vi "ISOP camera console.vi"() -> ()   [LabVIEW 2024]
uses:
  Global variables/global for picoscope.vi
  Global variables/Global for awg.vi
  Global variables/Global 1.vi
  Global variables/Global calib.vi
  Global variables/filepath global variable.vi
  <vilib>/Utility/file.llb/Write Delimited Spreadsheet (DBL).vi
  RIGOL DG4000 Series/RIGOL DG4000 Series.lvlib
  old LabVIEW files/labview_Mikami/Teledyne LeCroy WaveStation/Teledyne LeCroy WaveStation.lvlib
panel:
  in  "AOD exc λ2 [nm]":dbl=560.0
  in  "g2 monitor coeff [V/mdeg] am2":dbl=0.41
  in  "g1(SCAPE) phase":dbl=347.99999999999994
  in  "round-trip":bool
  in  "force":bool
  in  "vol rate [Hz]":dbl=123.00123001230013
  in  "vol period [s]":dbl=0.00813
  in  "xy pixsize [um]":dbl=0.4094999999999999
  in  "latest":bool=TRUE
  in  "g1 fit coeffs":path=path "E:/g1fitcalib/20241212-124823.g1fit"
  in  "?":bool
  in  "fit coeffs":dbl[][](array[numeric])=[[0.0003442175414953786, -6.156938994794033e-08], [-0.00558042162015375, 7.101515384977181e-07]]
  out "g2 ofst for calib":dbl=-0.1319999999999999 format="%_3g"
  in  "target freq for monitor":dbl=5.0
  in  "load config":bool
  in  "load config filepath":path
  in  "config filename":string
  in  "save config":bool
  in  "stop 2":bool
  in  "g1(scape)on/off":bool=TRUE
  in  "g1(SCAPE) p coeff":dbl format="%_4g"
  out "RIGOL name":refnum<visa-resource-name>="USB0::0x1AB1::0x0641::DG4E223801593::INSTR"
  in  "g1 (SCAPE) wvfm ofst [V]":dbl=1.0 format="%_4g"
  in  "g1 (SCAPE) gain adjust":dbl=1.0 format="%_4g"
  in  "g1 (SCAPE) gap adjust":dbl=1.0 format="%_4g"
  in  "rec with max freq":bool
  in  "target freq [Hz] for rec":dbl=10.0
  out "calib":bool
  in  "Config":T1={"Clock source"=enum."1200 MHz", "Active channel"=enum."Four channel", "Trigger direction"=enum."Positive (Rising edge)", "Trigger mode"=enum."Per trigger", "External Trigger enable"=TRUE, "Dac sample size"=enum."14 Bits LSB\n", "Dac sample format"=enum."Signed", "ClkDiv1"=2, "ClkDiv2"=1, "Output voltage \nlevel - Ch1"=1023, "Output voltage \nlevel - Ch2"=1023, "Output voltage\n level - Ch3"=1023, "Output voltage\n level - Ch4"=1023} {"Output voltage\n level - Ch4" min=1 max=1023 step=1 scale=0.0..1023.0; "Output voltage\n level - Ch3" min=1 max=1023 step=1 scale=0.0..1023.0; "Output voltage \nlevel - Ch2" min=1 max=1023 step=1 scale=0.0..1023.0; "Output voltage \nlevel - Ch1" min=1 max=1023 step=1 scale=0.0..1023.0}
  in  "AOD delay [us]":dbl
  in  "input to aod ch2 [mV]":dbl=680.0 min=0.0 max=2000.0
  in  "input to aod ch1 [mV]":dbl=280.0 min=0.0 max=2000.0
  out "REC":bool
  in  "Tdcam adj [us]":dbl=52.0
  in  "manual fast":bool
  in  "b adj":dbl format="%_3g"
  in  "Taod adjust [us]":dbl
  in  "BW adjust [MHz]":dbl=-13.0
  in  "dead time for burst [us]":dbl=30.0
  in  "g1 ofst":dbl format="%_3g"
  in  "g2 ofst":dbl=-0.1319999999999999 format="%_2g"
  in  "g1 monitor coeff [V/mdeg] am":dbl=0.5
  out "loop index":i32=43036
  out "g1 [Vpp]":dbl=0.4264766888294937
  out "g2 [Vpp]":dbl=3.79702857982119
  in  "g2 adj [%]":dbl=32.0
  in  "g1 (scape) adj [%]":dbl format="%#_3g"
  in  "FG3 (g1&g2) delay":dbl=60.0
  in  "g2 (img) phase":dbl=18.0 format="%_3g"
  in  "g2 sensitivity [V/mdeg] ao2":dbl=0.5
  in  "stop":bool
  out "Boolean":bool=TRUE
  out "g1 period [us]Tf1":dbl=3980.243621501115
  out "AOD BW [MHz] df":dbl=14.691598360655735
  out "FOV in z [um] FOVz":dbl=39.78847611827142
  in  "g1 sensitivity [V/mdeg] ao1":dbl=1.0
  in  "camera's pixel size [um] P":dbl=6.5
  out "AOD single scan time [us] Taod":dbl=42.30864503344067
  out "AOD scan interval [us] Tpp":dbl=139.51275699777062
  out "# of pixels in x Nx":dbl=141.32142857142858
  in  "pixels of camra line Ncam":dbl=2304.0
  in  "num of imgs per frame Nzf":dbl=16.0
  out "AOD delay [us] Tdaod":dbl=1457.5
  out "CAM delay [us] Tdcam":dbl=1272.0
  out "readout time [us] Tr":dbl=1440.0
  out "sym b":dbl=0.7530864197530864
  out "scan period [us] TL":dbl=2135.0
  in  "linear to full ratio of galvo g":dbl=0.7
  in  "min scan time [us] Tp2min":dbl=1000.0
  out "g2 period [us] Tf":dbl=4050.0
  in  "line readout time [us] tl":dbl=4.8
  in  "extra time for galvos [us]":dbl=110.0
  in  "AOD exc λ [nm]":dbl=488.0
  in  "AOD vel [m/s] vaod":dbl=4200.0
  in  "fex2":dbl=100.0
  in  "fex1":dbl=500.0
  in  "AOD anamo x mag":dbl=2.0
  in  "AOD anamo y mag":dbl=0.5
  out "M_tot":dbl=15.873015873015875
  in  "ft":dbl=100.0
  in  "f6":dbl=70.0
  in  "f5":dbl=100.0
  in  "f4":dbl=165.0
  in  "f3":dbl=70.0
  in  "f2":dbl=70.0
  in  "f1":dbl=165.0
  in  "ft_obj3":dbl=180.0
  in  "M_obj3":dbl=20.0
  in  "ft_obj2":dbl=180.0
  in  "M_obj2":dbl=20.0
  in  "ft_obj1":dbl=180.0
  in  "M_obj1":dbl=20.0
  in  "num of frames per vol Nv":dbl=2.0
  in  "z pixel size [um] pz":dbl=1.3
  in  "AOD scan speed ratio r":dbl=7.0
  in  "AOD power ratio Paod":dbl=1.0
  in  "exposure time [us] Tex":dbl=2500.0
  in  "num of voxels y Ny":dbl=300.0 min=4.0 max=2304.0 step=4.0
  # "for AOD"
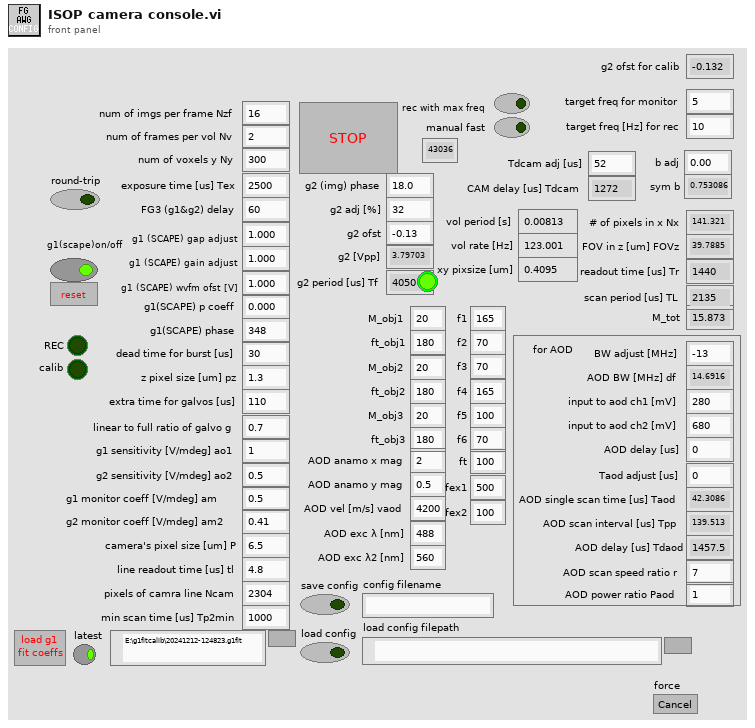
[diagram p1: front panel]
types:
  T1 = cluster{"Clock source":enum16{"1200 MHz", "900 MHz", "External"}, "Active channel":enum16{"Four channel", "Dual channel - Ch1 & Ch2", "Dual channel - Ch3 & Ch4", "Single channel - Ch1", "Single channel - Ch2", "Single channel - Ch3", "Single channel - Ch4"}, "Trigger direction":enum16{"Positive (Rising edge)", "Negative (Falling edge)"}, "Trigger mode":enum16{"Per trigger", "Continuous", "Single shot"}, "External Trigger enable":bool, "Dac sample size":enum16{"8 bits", "14 bits MSB", "14 Bits LSB\n"}, "Dac sample format":enum16{"Unsigned", "Signed"}, "ClkDiv1":u32, "ClkDiv2":u32, "Output voltage \nlevel - Ch1":u32, "Output voltage \nlevel - Ch2":u32, "Output voltage\n level - Ch3":u32, "Output voltage\n level - Ch4":u32}
  T2 = cluster{"BW [MHz]":dbl, "Taod [us]":dbl, "Nzf":i32, "Tpp [us]":dbl, "Tdaod [us]":dbl, "Tf2 [us]":dbl, "Nv":dbl, "ch1 range":dbl, "ch2 range":dbl, "wavel ratio":dbl, "delay [us]":dbl, "calib(F)/monitor(T)":bool}
  T3 = cluster{"b":dbl, "g":dbl, "Tf":dbl, "Tpp":dbl, "Nzf":dbl, "Nv":dbl, "pz":dbl, "g1toD":dbl, "agap":dbl, "again":dbl, "Vo":dbl}
  T4 = cluster{"waveform":dbl[], "Amplitude [Vpp]":dbl, "Frequency [Hz]":dbl}
  T5 = cluster{"g2 (img) phase":dbl, "x(1+0.01y)":dbl, "g2 ofst":dbl, "Vamp (p-p)":dbl, "Freq [Hz]":dbl, "g1(SCAPE) phase":dbl, "g1 (SCAPE) wvfm ofst [V]":dbl}
  T6 = cluster{"config":cluster{"BW [MHz]":dbl, "Taod [us]":dbl, "Nzf":i32, "Tpp [us]":dbl, "Tdaod [us]":dbl, "Tf2 [us]":dbl, "Nv":dbl, "ch1 range":dbl, "ch2 range":dbl, "wavel ratio":dbl, "delay [us]":dbl, "calib(F)/monitor(T)":bool}, "calib":bool}
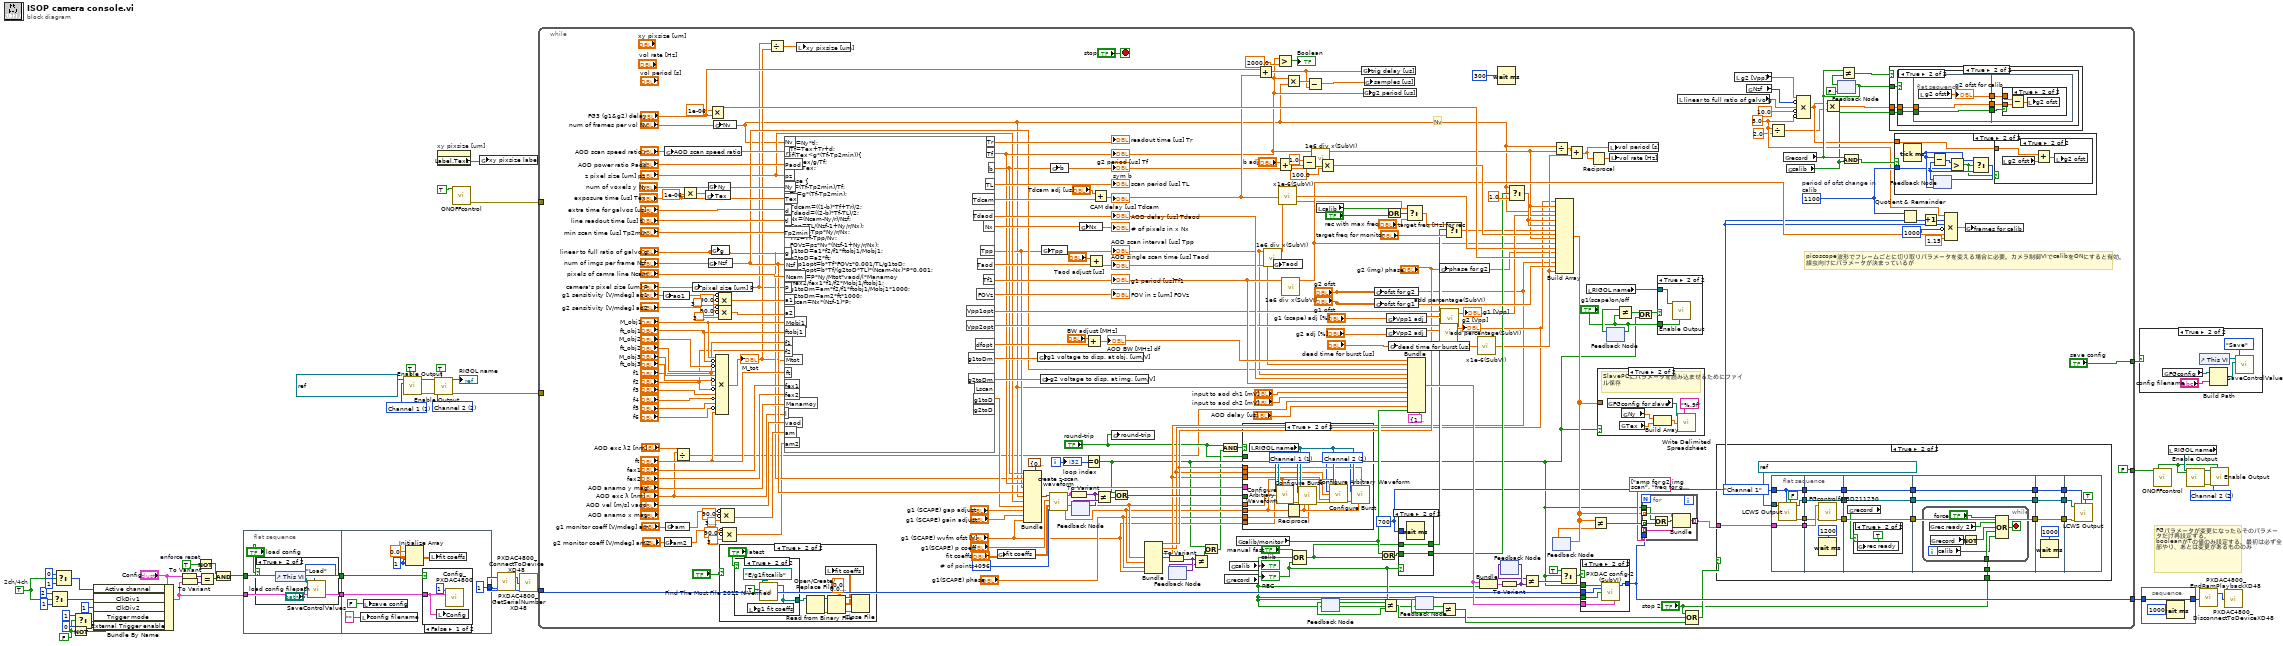
[diagram p0: block diagram]
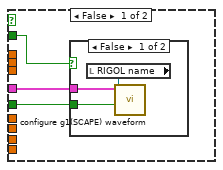
[diagram p5: hidden frame]
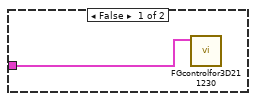
[diagram p7: hidden frame]
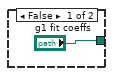
[diagram p10: hidden frame]
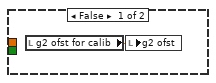
[diagram p12: hidden frame]
diagram:
  w2 = 2 items=["Channel 1"=1, "Channel 2"=2] ("Output Channel (1: Channel 1)")
  w5 = 1 items=["Channel 1"=1, "Channel 2"=2] ("Output Channel (1: Channel 1)")
  w6 = 2 items=["Channel 1"=1, "Channel 2"=2] ("Output Channel (1: Channel 1)")
  w35 = TRUE  # enforce reset
  w27 = FALSE ("continuous?")
  w28 = TRUE  # 2ch/4ch
  # "FGパラメータが変更になったらそのパラメータだけ再設定する。\nbooleanがTの値のみ設定する。最初は必ず全部やり、あとは変更があるもののみ"
  n1 = Select(t=u32 2 ("Value"), s=w28, f=u32 1 ("src_length_bytes")) -> (s? t:f=w40:u32)
  n2 = Select(t=u32 0 ("Value"), s=w28, f=u32 1 ("Value")) -> (s? t:f=w42:u32)
  n3 = Not(x=w27) -> (.not. x?=w36:bool)
  n4 = Select(t=u32 1 ("Value"), s=w27, f=u32 0 ("src_length_bytes")) -> (s? t:f=w37:u32)
  n5 = Bundle By Name(cluster="Config", "Active channel"=w42, "ClkDiv1"=w40, "ClkDiv2"=u32 1 ("src_length_bytes"), "Trigger mode"=w37, "External Trigger enable"=w36) -> (w26:T1)
  n6 = To Variant(anything="Config") -> (Variant=w24:variant)
  n7 = To Variant(anything=w26) -> (Variant=w23:variant)
  n8 = Not(x=w35) -> (.not. x?=w34:bool)
  n9 = Equal?(x=w24, y=w23) -> (x = y?=w22:bool)
  n10 = And(x=w34, y=w22) -> (x .and. y?=w33:bool)
  n11 = flat-sequence {
    tunnel: w26 -> [w49]
    tunnel: w33 -> [w50]
    tunnel: [w50] -> w14
    tunnel: [w49] -> w13
    tunnel: [u32 1 ("NumBoard")] -> w32
    tunnel: w14 -> [w61]
    tunnel: w13 -> [w59]
    frame #0 {
      n12 = case shown="True" "load config" {
        frame False {
        }
        frame True {
          n13 = control-ref of="This VI"() -> (w52:refnum<vi>)
          n14 = call "SaveControlValues.vi"("Mode"=enum16{"Save", "Load"}."Load" ("Save Control Values Mode"), "file path"="load config filepath", "Target VI"=w52) -> ()  [unwired: 2 in, 7 out]
        }
      }
    }
    frame #1 {
      w55 = 1 ("dimension size")
      n15 = local write "config filename"("" ("config filename")) -> ()
      n16 = local write "save config"(FALSE ("save config")) -> ()
      n17 = Initialize Array(0.0 ("element"), w55, w55) -> (w54:dbl[][])
      n18 = case shown="False" w61 {
        tunnel: w59 -> [w62 _]
        frame False {
          n19 = local write "Config"(w62) -> ()
          n20 = call "Config_PXDAC4800.vi"("NumBoard"=u32 1, "Config"=w62) -> ()  [unwired: 10 in, 4 out]
        }
        frame True {
        }
      }
      n21 = local write "fit coeffs"(w54) -> ()
    }
  }
  n22 = call "Enable Output.vi"("Enable Output (T: Enable)"=TRUE, "Output Channel (1: Channel 1)"=w5, "VISA resource name"=refnum<visa-resource-name> "USB0::0x1AB1::0x0641::DG4E223801593::INSTR") -> ("error out"=w8:errorcluster, "VISA resource name out"=w10:refnum<visa-resource-name>)  [unwired: 1 in, 6 out]
  n23 = call "Enable Output.vi"("Enable Output (T: Enable)"=TRUE, "error in (no error)"=w8, "Output Channel (1: Channel 1)"=w6, "VISA resource name"=w10) -> ("error out"=w7:errorcluster, "VISA resource name out"=→"RIGOL name":refnum<visa-resource-name>)  [unwired: 6 out]
  n24 = property on="xy pixsize [um]" class="DigNum (strict)"() -> ("Label.Text"=w12:string)  [unwired: 2 in, 2 out]
  n25 = call "ONOFFcontrol.vi"("Output ON/OFF (T: ON)"=TRUE) -> ("error out"=w47:errorcluster)  [unwired: 10 in]
  n26 = global write "filepath global variable.vi" "xy pixsize label"(w12) -> ()
  n27 = call "PXDAC4800_ConnectToDeviceXD48.vi"("brdNum"=w32) -> ("Handle Out"=w31:i64)  [unwired: 1 in, 1 out]
  n28 = call "PXDAC4800_GetSerialNumberXD48.vi"("Handle"=w31) -> ("Handle Out"=w21:i64)  [unwired: 2 out]
  n29 = while {
    tunnel: [FALSE ("Output ON/OFF (T: ON)")] -> w1
    tunnel: w47 -> [_]
    tunnel: w21 -> [w206]
    tunnel: [w204] -> w20
    tunnel: ["save config"] -> w15
    tunnel: w7 -> [_]
    i -> [w205]
    stop <- "stop" stop-if-true
    w117 = 4096  # # of points
    w134 = u32 700 ("milliseconds to wait")
    w142 = u32 1100  # period of ofst change in calib
    w124 = 5.0 ("value")
    # "picoscope波形でフレームごとに切り取りパラメータを変える場合に必要。カメラ制御VIでcalibをONにすると有効。\n線虫向けにパラメータが決まっているが"
    # "Nv"
    n30 = global write "global for picoscope.vi" "ao1"("g1 sensitivity [V/mdeg] ao1") -> ()
    n31 = global write "global for picoscope.vi" "am2"("g2 monitor coeff [V/mdeg] am2") -> ()
    n32 = global write "global for picoscope.vi" "AOD scan speed ratio"("AOD scan speed ratio r") -> ()
    n33 = global write "global for picoscope.vi" "am"("g1 monitor coeff [V/mdeg] am") -> ()
    n34 = Divide(x="AOD exc λ [nm]", y="AOD exc λ2 [nm]") -> (x/y=w64:dbl)
    n35 = Multiply(x=1e-06, y="exposure time [us] Tex") -> (x*y=w218:dbl)
    n36 = global write "global for picoscope.vi" "pixel size [um] P"("camera's pixel size [um] P") -> ()
    n37 = global write "Global for awg.vi" "Tex"(w218) -> ()
    n38 = global write "Global for awg.vi" "Ny"("num of voxels y Ny") -> ()
    n39 = global write "global for picoscope.vi" "Nzf"("num of imgs per frame Nzf") -> ()
    n40 = Multiply(x=1e-06, y="FG3 (g1&g2) delay") -> (x*y=w229:dbl)
    n41 = global write "global for picoscope.vi" "g"("linear to full ratio of galvo g") -> ()
    n42 = global write "global for picoscope.vi" "Nv"("num of frames per vol Nv") -> ()
    n43 = Compound Arithmetic op=MULTIPLY("M_obj1", invert "ft_obj1", invert "M_obj2", "ft_obj2", "M_obj3", invert "ft_obj3", "f1", invert "f2", "f3", invert "f4", "f5", invert "f6", "ft") -> (w109:dbl)
    "M_tot" <- w109
    n44 = Compound Arithmetic op=MULTIPLY(invert "g1 sensitivity [V/mdeg] ao1", invert 90.0 ("value"), 3.141592653589793) -> (w182:dbl)
    n45 = Compound Arithmetic op=MULTIPLY(invert "g2 sensitivity [V/mdeg] ao2", invert 90.0 ("value"), 3.141592653589793) -> (w181:dbl)
    n46 = case shown="True" "?" {
      frame False {
      }
      frame True {
        n47 = case shown="True" "latest" {
          tunnel: ["g1 fit coeffs" w356] -> w351
          frame False {
          }
          frame True {
            n48 = call "Find The Most File 2012 NIVerified.vi"("file(T)/folder(F)"=TRUE, "Folder Path In"=path "E:/g1fitcalib") -> ("File Path Out"=w356:path)  [unwired: 8 in, 1 out]
            n49 = local write "g1 fit coeffs"(w356) -> ()
          }
        }
        n50 = Open/Create/Replace File(file path (use dialog)=w351) -> (refnum out=w348:refnum<file>, error out=w350:errorcluster)  [unwired: 5 in, 1 out]
        n51 = Read from Binary File(5:dbl[][] [[0.0], [0.0], [0.0], [0.0], [0.0], [0.0], [0.0], [0.0], [0.0], [0.0], [0.0], [0.0], [0.0], [0.0], [0.0], [0.0], [0.0], [0.0], [0.0], [0.0], [0.0], [0.0], [0.0], [0.0], [0.0], [0.0], [0.0], [0.0], [0.0], [0.0], [0.0], [0.0], [0.0], [0.0], [0.0], [0.0], [0.0], [0.0], [0.0], [0.0], [0.0], [0.0], [0.0], [0.0], [0.0], [0.0], [0.0], [0.0], [0.0], [0.0], [0.0], [0.0], [0.0], [0.0], [0.0], [0.0], [0.0], [0.0], [0.0], [0.0], [0.0], [0.0], [0.0], [0.0], [0.0], [0.0], [0.0], [0.0], [0.0], [0.0], [0.0], [0.0], [0.0], [0.0], [0.0], [0.0], [0.0], [0.0], [0.0], [0.0], [0.0], [0.0], [0.0], [0.0], [0.0], [0.0], [0.0], [0.0], [0.0], [0.0], [0.0], [0.0], [0.0], [0.0], [0.0], [0.0], [0.0], [0.0], [0.0], [0.0], [0.0], [0.0], [0.0], [0.0], [0.0], [0.0], [0.0], [0.0], [0.0], [0.0], [0.0], [0.0], [0.0], [0.0], [0.0], [0.0], [0.0], [0.0], [0.0], [0.0], [0.0], [0.0], [0.0], [0.0], [0.0], [0.0], [0.0], [0.0], [0.0], [0.0], [0.0], [0.0], [0.0], [0.0], [0.0], [0.0], [0.0], [0.0], [0.0], [0.0], [0.0], [0.0], [0.0], [0.0], [0.0], [0.0], [0.0], [0.0], [0.0], [0.0], [0.0], [0.0], [0.0], [0.0], [0.0], [0.0], [0.0], [0.0], [0.0], [0.0], [0.0], [0.0], [0.0], [0.0], [0.0], [0.0], [0.0], [0.0], [0.0], [0.0], [0.0], [0.0], [0.0], [0.0], [0.0], [0.0], [0.0], [0.0], [0.0], [0.0], [0.0], [0.0], [0.0], [0.0], [0.0], [0.0], [0.0], [0.0], [0.0], [0.0], [0.0], [0.0], [0.0], [0.0], [0.0], [0.0], [0.0], [0.0], [0.0], [0.0], [0.0], [0.0], [0.0], [0.0], [0.0], [0.0], [0.0], [0.0], [0.0], [0.0], [0.0], [0.0], [0.0], [0.0], [0.0], [0.0], [0.0], [0.0], [0.0], [0.0], [0.0], [0.0], [0.0], [0.0], [0.0], [0.0], [0.0], [0.0], [0.0], [0.0], [0.0], [0.0], [0.0], [0.0], [0.0], [0.0], [0.0], [0.0], [0.0], [0.0], [0.0], [0.0], [0.0], [0.0], [0.0], [0.0], [0.0], [0.0], [0.0], [0.0], [0.0], [0.0], [0.0], [0.0], [0.0], [0.0]] ("fit coeffs"), 8:w350, 11:w348) -> (0:w349:errorcluster, 2:w346:dbl[][], 3:w347:refnum<file>)  [unwired: 3 in, 1 out]
        n52 = local write "fit coeffs"(w346) -> ()
        n53 = Close File(refnum=w347, error in=w349) -> ()  [unwired: 2 out]
      }
    }
    n54 = Compound Arithmetic op=MULTIPLY(invert "g1 monitor coeff [V/mdeg] am", invert 90.0 ("value"), 3.141592653589793) -> (w171:dbl)
    n55 = Compound Arithmetic op=MULTIPLY(invert "g2 monitor coeff [V/mdeg] am2", invert 90.0 ("value"), 3.141592653589793) -> (w67:dbl)
    n56 = Divide(x="camera's pixel size [um] P", y=w109) -> (x/y=w107:dbl)
    n57 = formula code="Tr=Ny*tl;\nTf=Tex+Tr+d;\nif(Tex<g*(Tf-Tp2min)){\nb=Tex/g/Tf;\nTL=Tex;\n} \nelse {\nb=(Tf-Tp2min)/Tf;\nTL=g*(Tf-Tp2min);\n}\nTdcam=((1-b)*Tf+Tr)/2;\nTdaod=((2-b)*Tf-TL)/2;\nNx=(Ncam-Ny/r)/Nzf;\nTpp=TL/(Nzf-1+Ny/r/Nx);\nTaod=Tpp*Ny/r/Nx;\nTf1=Tf-Tpp/Nv;\nFOVz=pz*Nv*(Nzf-1+Ny/r/Nx);\ng1toD=a1*f2/f1*ftobj1/Mobj1;\ng2toD=a2*ft;\nVpp1opt=b*Tf*FOVz*0.001/TL/g1toD;\nVpp2opt=b*Tf/(g2toD*TL)*(Ncam-Nx)*P*0.001;\ndfopt=P*Ny/Mtot*vaod/l*Manamoy\n*fex2/fex1*f1/f2*Mobj1/ftobj1;\ng1toDm=am*f2/f1*ftobj1/Mobj1*1000;\ng2toDm=am2*ft*1000;\nLscan=Nx*(Nzf-1)*P;"("Nv"="num of frames per vol Nv", "r"="AOD scan speed ratio r", "Paod"="AOD power ratio Paod", "pz"="z pixel size [um] pz", "Ny"="num of voxels y Ny", "Tex"="exposure time [us] Tex", "Mtot"=w109, "d"="extra time for galvos [us]", "tl"="line readout time [us] tl", "Tp2min"="min scan time [us] Tp2min", "g"="linear to full ratio of galvo g", "Nzf"="num of imgs per frame Nzf", "Ncam"="pixels of camra line Ncam", "P"="camera's pixel size [um] P", "a1"=w182, "ft"="ft", "Mobj1"="M_obj1", "ftobj1"="ft_obj1", "f1"="f1", "f2"="f2", "vaod"="AOD vel [m/s] vaod", "Manamoy"="AOD anamo y mag", "fex1"="fex1", "fex2"="fex2", "l"="AOD exc λ [nm]", "a2"=w181, "am"=w171, "am2"=w67) -> ("Tf"=w169:dbl, "Tr"=→"readout time [us] Tr":dbl, "b"=w115:dbl, "TL"=→"scan period [us] TL":dbl, "Tdcam"=w211:dbl, "Tdaod"=w210:dbl, "Nx"=w231:dbl, "Tpp"=w114:dbl, "Taod"=w241:dbl, "FOVz"=→"FOV in z [um] FOVz":dbl, "Vpp1opt"=w191:dbl, "Vpp2opt"=w192:dbl, "dfopt"=w242:dbl, "Tf1"=w221:dbl, "g1toDm"=w235:dbl, "g2toDm"=w234:dbl, "g1toD"=w166:dbl)  [unwired: 2 out]
    "g2 period [us] Tf" <- w169
    "sym b" <- w115
    "AOD delay [us] Tdaod" <- w210
    "# of pixels in x Nx" <- w231
    "AOD scan interval [us] Tpp" <- w114
    "g1 period [us]Tf1" <- w221
    n58 = local write "xy pixsize [um]"(w107) -> ()
    n59 = global write "global for picoscope.vi" "fit coeffs"("fit coeffs") -> ()
    n60 = Bundle(cluster=T3 {"b"=0.5, "g"=0.7, "Tf"=2500.0, "Tpp"=58.0, "Nzf"=16.0, "Nv"=8.0, "pz"=1.3, "g1toD"=0.13328, "agap"=1.0, "again"=1.0, "Vo"=1.0} ("input"), "b"=w115, "g"="linear to full ratio of galvo g", "Tf"=w169, "Tpp"=w114, "Nzf"="num of imgs per frame Nzf", "Nv"="num of frames per vol Nv", "pz"="z pixel size [um] pz", "g1toD"=w166, "agap"="g1 (SCAPE) gap adjust", "again"="g1 (SCAPE) gain adjust", "Vo"="g1 (SCAPE) wvfm ofst [V]") -> (w86:T3)
    n61 = global write "global for picoscope.vi" "g1 voltage to disp. at obj. [um/V]"(w235) -> ()
    n62 = global write "global for picoscope.vi" "g2 voltage to disp. at img. [um/V]"(w234) -> ()
    n63 = global write "global for picoscope.vi" "Tpp"(w114) -> ()
    n64 = call "create z-scan waveform.vi"("# of points"=w117, "fit coeffs"="fit coeffs", "parabollic coeff"="g1(SCAPE) p coeff", "input"=w86) -> ("Freq [Hz]"=w81:dbl, "Vamp (p-p)"=w82:dbl, "output cluster"=w160:T4)  [unwired: 5 in]
    n65 = global write "global for picoscope.vi" "b"(w115) -> ()
    n66 = To Variant(anything=w160) -> (Variant=w162:variant)
    n67 = feedback #1() -> (w163:variant)  [unwired: 1 in]
    n68 = feedback-in #1(w162) -> ()
    n69 = global write "global for picoscope.vi" "Nx"(w231) -> ()
    n70 = Equal To 0?(x=w205) -> (x = 0?=w74:bool)
    n71 = Add(x="BW adjust [MHz]", y=w242) -> (x+y=w222:dbl)
    "AOD BW [MHz] df" <- w222
    n72 = Add(x="Taod adjust [us]", y=w241) -> (x+y=w118:dbl)
    "AOD single scan time [us] Taod" <- w118
    n73 = Add(x="Tdcam adj [us]", y=w211) -> (x+y=w193:dbl)
    "CAM delay [us] Tdcam" <- w193
    n74 = Not Equal?(x=w162, y=w163) -> (x != y?=w161:bool)
    n75 = global write "global for picoscope.vi" "round-trip"("round-trip") -> ()
    n76 = Or(x=w74, y=w161) -> (x .or. y?=w159:bool)
    n77 = feedback #2() -> (w76:variant)  [unwired: 1 in]
    n78 = global read "Global 1.vi" "record"() -> (w92:bool)
    "REC" <- w92
    n79 = global read "Global calib.vi" "calib"() -> (w87:bool)
    "calib" <- w87
    n80 = global read "global for picoscope.vi" "calib/monitor"() -> (w145:bool)
    n81 = Add(x="FG3 (g1&g2) delay", y=w193) -> (x+y=w238:dbl)
    n82 = call "1e6 div x(SubVI).vi"("x"=w114) -> ("1e6/x"=w105:dbl)  [unwired: 10 in]
    n83 = global write "global for picoscope.vi" "Taod"(w118) -> ()
    n84 = Greater?(x=w169, y=2000.0) -> (0:→"Boolean":bool)
    n85 = Add(x="b adj", y=w115) -> (x+y=w214:dbl)
    n86 = call "x1e-6(SubVI).vi"("in"=w193) -> ("out"=w194:dbl)
    n87 = call "1e6 div x(SubVI).vi"("x"=w221) -> ("1e6/x"=w138:dbl)  [unwired: 10 in]
    n88 = Multiply(x=w169, y="num of frames per vol Nv") -> (x*y=w239:dbl)
    n89 = Compound Arithmetic op=OR("manual fast", w87, w92) -> (w106:bool)
    n90 = Subtract(x=1.0, y=w214) -> (x-y=w247:dbl)
    n91 = Subtract(x=w239, y=w238) -> (x-y=w237:dbl)
    n92 = call "1e6 div x(SubVI).vi"("x"=w169) -> ("1e6/x"=w102:dbl)  [unwired: 10 in]
    n93 = local read "calib"() -> (w96:bool)
    n94 = Multiply(x=w247, y=100.0) -> (x*y=w230:dbl)
    n95 = feedback #3() -> (w93:bool)  [unwired: 1 in]
    n96 = feedback-in #3(w92) -> ()
    n97 = global write "global for picoscope.vi" "trig delay [us]"(w238) -> ()
    n98 = global write "global for picoscope.vi" "g2 period [us]"(w169) -> ()
    n99 = global write "global for picoscope.vi" "samples [us]"(w237) -> ()
    n100 = global write "global for picoscope.vi" "ofst for g2"("g2 ofst") -> ()
    n101 = global write "global for picoscope.vi" "ofst for g1"("g1 ofst") -> ()
    n102 = Or(x=w145, y=w106) -> (x .or. y?=w149:bool)
    n103 = Not Equal?(x=w92, y=w93) -> (x != y?=w90:bool)
    n104 = Or(x=w96, y="rec with max freq") -> (x .or. y?=w94:bool)
    n105 = global write "global for picoscope.vi" "Vpp1 adj"("g1 (scape) adj [%]") -> ()
    n106 = global write "global for picoscope.vi" "Vpp2 adj"("g2 adj [%]") -> ()
    n107 = global write "global for picoscope.vi" "dead time for burst [us]"("dead time for burst [us]") -> ()
    n108 = case shown="True" w92 {
      tunnel: [w399 w402] -> w148
      tunnel: w149 -> [w399 w402]
      tunnel: w106 -> [w398 w401]
      tunnel: [w398 w401] -> w144
      tunnel: w134 -> [_ w400]
      frame False {
      }
      frame True {
        n109 = Wait (ms)(milliseconds to wait=w400) -> ()  [unwired: 1 out]
      }
    }
    n110 = Select(t=w105, s=w94, f="target freq [Hz] for rec") -> (s? t:f=w103:dbl)
    n111 = Bundle(cluster=T2 {"BW [MHz]"=19.691598360655735, "Taod [us]"=29.10737386804657, "Nzf"=5, "Tpp [us]"=217.72315653298836, "Tdaod [us]"=1357.142857142857, "Tf2 [us]"=2395.569210866753, "Nv"=4.0, "ch1 range"=580.0, "ch2 range"=680.0, "wavel ratio"=0.871, "delay [us]"=-40.0, "calib(F)/monitor(T)"=FALSE} ("config"), "BW [MHz]"=w222, "Taod [us]"=w118, "Nzf"="num of imgs per frame Nzf", "Tpp [us]"=w114, "Tdaod [us]"=w210, "Tf2 [us]"=w221, "Nv"="num of frames per vol Nv", "ch1 range"="input to aod ch1 [mV]", "ch2 range"="input to aod ch2 [mV]", "wavel ratio"=w64, "delay [us]"="AOD delay [us]", "calib(F)/monitor(T)"=w145) -> (w200:T2)
    n112 = feedback #4() -> (w157:bool)  [unwired: 1 in]
    n113 = feedback-in #4(w87) -> ()
    n114 = global write "global for picoscope.vi" "phase for g2"("g2 (img) phase") -> ()
    n115 = call "add percentage(SubVI).vi"("y%"="g2 adj [%]", "x"=w192) -> ("x(1+0.01y)"=w84:dbl)  [unwired: 3 in]
    "g2 [Vpp]" <- w84
    n116 = Bundle("g2 (img) phase"="g2 (img) phase", "x(1+0.01y)"=w84, "g2 ofst"="g2 ofst", "Vamp (p-p)"=w82, "Freq [Hz]"=w81, "g1(SCAPE) phase"="g1(SCAPE) phase", "g1 (SCAPE) wvfm ofst [V]"="g1 (SCAPE) wvfm ofst [V]") -> (w77:T5)  [unwired: 1 in]
    n117 = To Variant(anything=w77) -> (Variant=w78:variant)
    n118 = feedback-in #2(w78) -> ()
    n119 = Not Equal?(x=w78, y=w76) -> (x != y?=w73:bool)
    n120 = Or(x=w74, y=w73) -> (x .or. y?=w72:bool)
    n121 = And(x="round-trip", y=w72) -> (x .and. y?=w75:bool)
    n122 = case shown="True" w75 {
      tunnel: w160 -> [w270 _]
      tunnel: w159 -> [w269 _]
      tunnel: w82 -> [_ w287]
      tunnel: w81 -> [_ w282]
      tunnel: "g2 (img) phase" -> [_ w279]
      tunnel: w84 -> [_ w278]
      tunnel: "g2 ofst" -> [_ w277]
      tunnel: "g1(SCAPE) phase" -> [_ w276]
      tunnel: "g1 (SCAPE) wvfm ofst [V]" -> [_ w274]
      tunnel: "round-trip" -> [w268 _]
      frame False {
        n123 = case shown="False" w268 {
          tunnel: w270 -> [w272 _]
          tunnel: w269 -> [w271 _]
          frame False {
            n124 = local read "RIGOL name"() -> (w273:refnum<visa-resource-name>)
            n125 = call "configure g1(SCAPE) waveform.vi"("VISA resource name"=w273, "enable"=w271, "output cluster"=w272) -> ()  [unwired: 8 in, 1 out]
          }
          frame True {
          }
        }
      }
      frame True {
        w275 = 2 items=["Channel 1"=1, "Channel 2"=2] ("Output Channel (1: Channel 1)")
        w285 = 1 items=["Channel 1"=1, "Channel 2"=2] ("Output Channel (1: Channel 1)")
        n126 = local read "RIGOL name"() -> (w284:refnum<visa-resource-name>)
        n127 = call "Configure Arbitrary Waveform.vi"("VISA resource name"=w284, "Frequency (1000 Hz)"=w282, "Output Channel (1: Channel 1)"=w285, "Amplitude (5 Vpp)"=w287, "Offset (0)"=w274) -> ("error out"=w286:errorcluster)  [unwired: 9 in, 1 out]
        n128 = Reciprocal(x=w282) -> (1/x=w283:dbl)
        n129 = call "Configure Burst.vi"("VISA resource name"=w284, "Burst Channel (1: Channel 1)"=w285, "error in (no error)"=w286, "Burst Period (0.01 s)"=w283, "Start Phase (0 degree)"=w276) -> ("error out"=w281:errorcluster)  [unwired: 9 in, 1 out]
        n130 = call "Configure Arbitrary Waveform.vi"("VISA resource name"=w284, "Frequency (1000 Hz)"=w282, "Output Channel (1: Channel 1)"=w275, "Amplitude (5 Vpp)"=w278, "error in (no error)"=w281, "Offset (0)"=w277) -> ("error out"=w280:errorcluster)  [unwired: 8 in, 1 out]
        n131 = call "Configure Burst.vi"("VISA resource name"=w284, "Burst Channel (1: Channel 1)"=w275, "error in (no error)"=w280, "Burst Period (0.01 s)"=w283, "Start Phase (0 degree)"=w279) -> ()  [unwired: 9 in, 2 out]
      }
    }
    n132 = Not Equal?(x=w87, y=w157) -> (x != y?=w156:bool)
    n133 = call "add percentage(SubVI).vi"("y%"="g1 (scape) adj [%]", "x"=w191) -> ("x(1+0.01y)"=w189:dbl)  [unwired: 3 in]
    "g1 [Vpp]" <- w189
    n134 = Select(t=w103, s=w144, f="target freq for monitor") -> (s? t:f=w147:dbl)
    n135 = call "x1e-6(SubVI).vi"("in"="dead time for burst [us]") -> ("out"=w99:dbl)
    n136 = Bundle("config"=w200, "calib"=w87) -> (w199:T6)  [unwired: 1 in]
    n137 = Wait (ms)(milliseconds to wait=300) -> ()  [unwired: 1 out]
    n138 = feedback #5() -> (w196:variant)  [unwired: 1 in]
    n139 = To Variant(anything=w199) -> (Variant=w197:variant)
    n140 = feedback-in #5(w197) -> ()
    n141 = Select(t="num of frames per vol Nv", s=w148, f=1.0 ("t")) -> (s? t:f=w216:dbl)
    n142 = Not Equal?(x=w196, y=w197) -> (x != y?=w203:bool)
    n143 = Divide(x="num of frames per vol Nv", y=w102) -> (x/y=w100:dbl)
    n144 = feedback #6() -> (w186:dbl[])  [unwired: 1 in]
    n145 = Build Array(w84, w102, "num of frames per vol Nv", w189, w216, w216, w147, w230, w102, w138, w194, "g2 (img) phase", w229, "g2 ofst", "g1 ofst", w99) -> (w187:dbl[])
    n146 = feedback-in #6(w187) -> ()
    n147 = Select(t=TRUE, s=w74, f=w203) -> (s? t:f=w198:bool)
    n148 = Add(x=w100, y=w99) -> (x+y=w97:dbl)
    n149 = case shown="True" w198 {
      tunnel: w206 -> [w387 w392]
      tunnel: [w387 w391] -> w204
      tunnel: w74 -> [_ w390]
      tunnel: w200 -> [_ w388]
      tunnel: w87 -> [_ w389]
      frame False {
      }
      frame True {
        n150 = call "PXDAC config-2 (SubVI).vi"("Handle Out in"=w392, "first run?"=w390, "calib (no out to AWG)"=w389, "config"=w388) -> ("Handle Out out"=w391:i64)  [unwired: 9 in, 2 out]
      }
    }
    n151 = local read "RIGOL name"() -> (w155:refnum<visa-resource-name>)
    n152 = Reciprocal(x=w97) -> (1/x=w98:dbl)
    n153 = Not Equal?(x=w187, y=w186) -> (x != y?=w227:bool[])
    n154 = case shown="True" w74 {
      tunnel: w187 -> [_ _]
      frame False {
      }
      frame True {
        # "SlavePCにパラメータを読み込ませるためにファイル保存"
        n155 = global read "filepath global variable.vi" "FGconfig for slave"() -> (w393:path)
        n156 = global read "Global for awg.vi" "Tex"() -> (w396:dbl)
        n157 = global read "Global for awg.vi" "Ny"() -> (w397:dbl)
        n158 = Build Array(w397, w396) -> (w395:dbl[])
        n159 = call-poly <vilib>:"Write Delimited Spreadsheet.vi"("file path (dialog if empty)"=w393, "format (%.3f)"="%.9f", "1D data"=w395) -> ()  [unwired: 11 in, 2 out]
      }
    }
    n160 = feedback #7() -> (w153:bool)  [unwired: 1 in]
    n161 = feedback-in #7("g1(scape)on/off") -> ()
    n162 = local write "vol period [s]"(w97) -> ()
    n163 = local write "vol rate [Hz]"(w98) -> ()
    n164 = Not Equal?(x=w153, y="g1(scape)on/off") -> (x != y?=w154:bool)
    n165 = Or(x=w154, y=w74) -> (x .or. y?=w119:bool)
    n166 = for {
      tunnel: w227 -> [w404] mode=indexing
      tunnel: w187 -> [w408] mode=indexing
      tunnel: [w407] -> w91 mode=indexing
      tunnel: string[] ["amp for g2 img scan", "freq for g2 (img scan)", "cycs for 3D scan", "amp for g1 (scape)", "cycs for awg", "delay for awg", "freq for awg2", "sym for g1g2", "freq for awg1", "freq for g1 (scape)", "delay for cam", "phase for g2 (img scan)", "delay for FG3 (awg&cam)", "ofst for g2 (img scan)", "ofst for g1 (scape)", "dead time for burst"] -> [w406] mode=indexing
      tunnel: w74 -> [w405]
      tunnel: w204 -> [_]
      n167 = Or(x=w405, y=w404) -> (x .or. y?=w403:bool)
      n168 = Bundle("out"=w408, w403, w406) -> (w407:cluster{"out":dbl, bool, string})  [unwired: 1 in]
    }
    n169 = case shown="True" w119 {
      tunnel: w155 -> [_ w386]
      tunnel: "g1(scape)on/off" -> [_ w385]
      frame False {
      }
      frame True {
        n170 = call "Enable Output.vi"("Enable Output (T: Enable)"=w385, "VISA resource name"=w386) -> ()  [unwired: 2 in, 8 out]
      }
    }
    n171 = local read "linear to full ratio of galvo g"() -> (w127:dbl)
    n172 = Compound Arithmetic op=OR("stop 2", w90, w156) -> (w89:bool)
    n173 = case shown="True" w89 {
      tunnel: w91 -> [w288 w302]
      tunnel: "stop 2" -> [_ w295]
      frame False {
        n174 = call "FGcontrolfor3D211230.vi"("Array 3"=w288) -> ()  [unwired: 7 in, 4 out]
      }
      frame True {
        n175 = flat-sequence {
          tunnel: refnum<visa-resource-name> "USB0::0x05FF::0x0A21::LCRY2362C01698::INSTR" ("VISA resource name") -> [w310]
          tunnel: enum16{"Channel 1", "Channel 2"}."Channel 1" ("Channel (1)") -> [w313]
          tunnel: [w313] -> w308
          tunnel: [w312] -> w307
          tunnel: [w311] -> w306
          tunnel: [w309] -> w305
          tunnel: w302 -> [w309]
          tunnel: w308 -> [w320]
          tunnel: [w320] -> w301
          tunnel: w307 -> [w319]
          tunnel: [w319] -> w300
          tunnel: [w316] -> w299
          tunnel: w306 -> [w315]
          tunnel: w305 -> [w317]
          tunnel: w301 -> [w324]
          tunnel: [w324] -> w298
          tunnel: w300 -> [w323]
          tunnel: [w323] -> w297
          tunnel: w299 -> [w322]
          tunnel: [w322] -> w296
          tunnel: w298 -> [w329]
          tunnel: [w329] -> w294
          tunnel: w297 -> [w328]
          tunnel: [w328] -> w292
          tunnel: w296 -> [w327]
          tunnel: [w327] -> w290
          tunnel: w295 -> [w326]
          tunnel: w294 -> [w340]
          tunnel: [w340] -> w293
          tunnel: w292 -> [w339]
          tunnel: [w339] -> w291
          tunnel: w290 -> [w338]
          tunnel: [w338] -> w289
          tunnel: w293 -> [w343]
          tunnel: w291 -> [w342]
          tunnel: w289 -> [w341]
          frame #0 {
            n176 = call "LCWS Output.vi"("Output ON/OFF (T: ON)"=FALSE, "Channel (1)"=w313, "VISA resource name"=w310) -> ("error out"=w311:errorcluster, "VISA resource name out"=w312:refnum<visa-resource-name>)  [unwired: 7 in]
          }
          frame #1 {
            n177 = call "FGcontrolfor3D211230.vi"("error in (no error)"=w315, "Array 3"=w317) -> ("error out"=w316:errorcluster)  [unwired: 6 in, 3 out]
            n178 = Wait (ms)(milliseconds to wait=u32 1200) -> ()  [unwired: 1 out]
          }
          frame #2 {
            n179 = global read "Global 1.vi" "record"() -> (w321:bool)
            n180 = case shown="True" w321 {
              frame False {
              }
              frame True {
                n181 = global write "Global 1.vi" "rec ready"(TRUE ("rec ready")) -> ()
              }
            }
          }
          frame #3 {
            n182 = while {
              tunnel: w326 -> [w331]
              stop <- w335 stop-if-true
              n183 = global read "Global 1.vi" "rec ready 2"() -> (w336:bool)
              n184 = global read "Global 1.vi" "record"() -> (w333:bool)
              n185 = global read "Global calib.vi" "calib"() -> (w330:bool)
              n186 = Not(x=w333) -> (.not. x?=w332:bool)
              n187 = Compound Arithmetic op=OR("force", w336, w332, w331, w330) -> (w335:bool)
            }
          }
          frame #4 {
            n188 = Wait (ms)(milliseconds to wait=u32 1000 ("millisecond timer value")) -> ()  [unwired: 1 out]
          }
          frame #5 {
            n189 = call "LCWS Output.vi"("Output ON/OFF (T: ON)"=TRUE, "Channel (1)"=w343, "error in (no error)"=w341, "VISA resource name"=w342) -> ()  [unwired: 6 in, 2 out]
          }
        }
      }
    }
    n190 = local read "g2 [Vpp]"() -> (w129:dbl)
    n191 = global read "global for picoscope.vi" "Nzf"() -> (w128:i32)
    n192 = Divide(x=w124, y=2.0) -> (x/y=w122:dbl)
    n193 = global read "Global 1.vi" "record"() -> (w130:bool)
    n194 = global read "Global 1.vi" "calib"() -> (w120:bool)
    n195 = Compound Arithmetic op=MULTIPLY(w129, invert w128, w127, invert 10.0 ("value"), invert w124) -> (w125:dbl)
    n196 = Multiply(x=w125, y=w122) -> (x*y=w121:dbl)
    n197 = feedback #8(FALSE ("record")) -> (w133:bool)
    n198 = feedback-in #8(w130) -> ()
    n199 = Not Equal?(x=w130, y=w133) -> (x != y?=w131:bool)
    n200 = And(x=w130, y=w120) -> (x .and. y?=w143:bool)
    n201 = case shown="True" w131 {
      tunnel: w130 -> [_ w359]
      tunnel: w121 -> [_ w358]
      tunnel: w120 -> [_ w357]
      frame False {
      }
      frame True {
        n202 = case shown="True" w359 {
          tunnel: w358 -> [_ w364]
          tunnel: w357 -> [_ w362]
          frame False {
            n203 = local read "g2 ofst for calib"() -> (w360:dbl)
            n204 = local write "g2 ofst"(w360) -> ()
          }
          frame True {
            n205 = flat-sequence {
              tunnel: [w368] -> w365
              tunnel: w364 -> [w367]
              tunnel: [w367] -> w363
              tunnel: w362 -> [w366]
              tunnel: [w366] -> w361
              tunnel: w365 -> [w371]
              tunnel: w363 -> [w370]
              tunnel: w361 -> [w369]
              frame #0 {
                n206 = local read "g2 ofst"() -> (w368:dbl)
                "g2 ofst for calib" <- w368
              }
              frame #1 {
                n207 = case shown="True" w369 {
                  tunnel: w371 -> [_ w374]
                  tunnel: w370 -> [_ w373]
                  frame False {
                  }
                  frame True {
                    n208 = Subtract(x=w374, y=w373) -> (x-y=w372:dbl)
                    n209 = local write "g2 ofst"(w372) -> ()
                  }
                }
              }
            }
          }
        }
      }
    }
    n210 = case shown="True" w143 {
      tunnel: w142 -> [_ w376]
      tunnel: w125 -> [_ w375]
      frame False {
      }
      frame True {
        n211 = Tick Count (ms)() -> (millisecond timer value=w378:u32)
        n212 = feedback #9(w378) -> (w380:u32)
        n213 = Subtract(x=w378, y=w380) -> (x-y=w381:u32)
        n214 = Greater?(x=w381, y=w376) -> (0:w377:bool)
        n215 = Select(t=w378, s=w377, f=w380) -> (s? t:f=w379:u32)
        n216 = feedback-in #9(w379) -> ()
        n217 = case shown="True" w377 {
          tunnel: w375 -> [_ w382]
          frame False {
          }
          frame True {
            n218 = local read "g2 ofst"() -> (w383:dbl)
            n219 = Add(x=w382, y=w383) -> (x+y=w384:dbl)
            n220 = local write "g2 ofst"(w384) -> ()
          }
        }
      }
    }
    n221 = Quotient & Remainder(x=w142, y=w134) -> (floor(x/y)=w141:u32)  [unwired: 1 out]
    n222 = Increment(x=w141) -> (x+1=w135:u32)
    n223 = Compound Arithmetic op=MULTIPLY(w124, w135, w134, invert 1000 ("value"), w138, 1.15 ("value")) -> (w137:dbl)
    n224 = global write "global for picoscope.vi" "frames for calib"(w137) -> ()
    "loop index" <- w205
  }
  n225 = case shown="True" w15 {
    frame False {
    }
    frame True {
      n226 = global read "filepath global variable.vi" "FGconfig"() -> (w409:path)
      n227 = control-ref of="This VI"() -> (w413:refnum<vi>)
      n228 = Build Path(base path=w409, name or relative path="config filename") -> (appended path=w410:path)
      n229 = call "SaveControlValues.vi"("Mode"=enum16{"Save", "Load"}."Save" ("Save Control Values Mode"), "file path"=w410, "Target VI"=w413) -> ()  [unwired: 2 in, 7 out]
    }
  }
  n230 = stacked-sequence {
    tunnel: [w414] -> w30
    tunnel: w20 -> [w414]
    frame #0 {
      n231 = Wait (ms)(milliseconds to wait=1000) -> ()  [unwired: 1 out]
    }
  }
  n232 = call "ONOFFcontrol.vi"("Output ON/OFF (T: ON)"=w1) -> ()  [unwired: 10 in, 1 out]
  n233 = local read "RIGOL name"() -> (w16:refnum<visa-resource-name>)
  n234 = call "Enable Output.vi"("Enable Output (T: Enable)"=w1, "VISA resource name"=w16) -> ("error out"=w3:errorcluster, "VISA resource name out"=w4:refnum<visa-resource-name>)  [unwired: 2 in, 6 out]
  n235 = call "PXDAC4800_EndRamPlaybackXD48.vi"("Handle"=w30) -> ("Handle out"=w29:i64)  [unwired: 1 out]
  n236 = call "Enable Output.vi"("Enable Output (T: Enable)"=w1, "error in (no error)"=w3, "Output Channel (1: Channel 1)"=w2, "VISA resource name"=w4) -> ()  [unwired: 8 out]
  n237 = call "PXDAC4800_DisconnectToDeviceXD48.vi"("Handle"=w29) -> ()  [unwired: 1 out]
